vi "AES New.vi"(8 "error in (no error)":errorcluster, 9 "mode":i32(ring)=1 items=["CBC"=1, "ECB"=2, "OFB"=3, "CFB"=4, "CTS"=5], 10 "block size":i32=128, 11 "key size":i32=256) -> (0 "error out":errorcluster, 3 "AES out":refnum<class "AES.lvclass">)   [LabVIEW 2021, in "AES.lvclass"]
uses:
  AES.lvclass
  AES.lvclass/AES.ctl
  System.Core
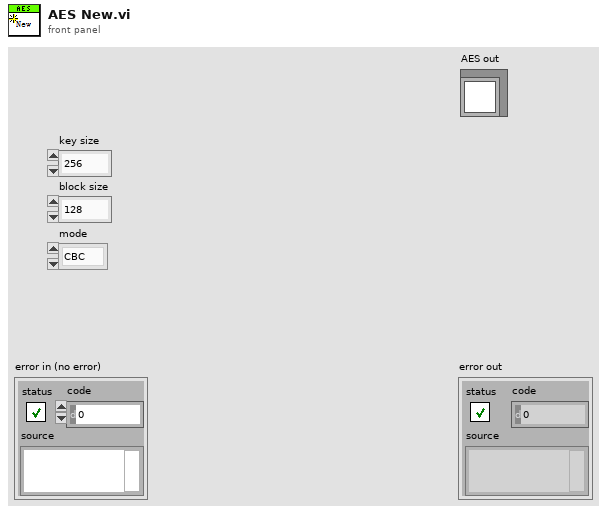
[diagram p1: front panel]
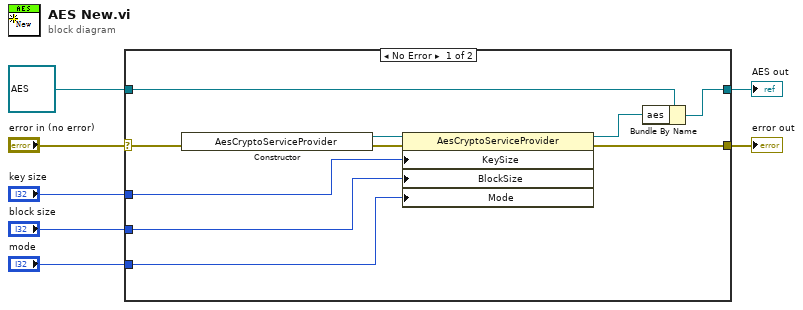
[diagram p0: block diagram]
diagram:
  n1 = case shown="No Error" "error in (no error)" {
    selector: "error in (no error)" -> [w15 w19]
    tunnel: [w14 w19] -> w6
    tunnel: [w11 w18] -> w4
    tunnel: refnum<class "AES.lvclass"> refnum ("AES in") -> [w13 w18]
    tunnel: "key size" -> [w10 _]
    tunnel: "block size" -> [w9 _]
    tunnel: "mode" -> [w8 _]
    frame No Error {
      n2 = constructor class="AesCryptoServiceProvider" ("AliceEntschlüsselt")(error in=w15) -> (reference out=w16:refnum<k24>, error out=w17:errorcluster)  [unwired: 2 in, 1 out]
      n3 = property class="AesCryptoServiceProvider"(reference=w16, error in=w17, "KeySize"=w10, "BlockSize"=w9, "Mode"=w8) -> (reference out=w12:refnum<k24>, error out=w14:errorcluster)
      n4 = Bundle By Name(cluster=w13, "aes"=w12) -> (w11:refnum<class "AES.lvclass">)
    }
    frame Error {
    }
  }
  "error out" <- w6
  "AES out" <- w4
